vi "robot main.vi"() -> ()   [LabVIEW 2012]
uses:
  <vilib>/robotics/Starter Kit/1.0/9631 Host Interface/NI_Robotics_Starter Kit Host_9631_1.0.lvclass
  <vilib>/robotics/Starter Kit/Host Interface/NI_Robotics_Starter Kit Host.lvclass
panel:
  in  "stop":bool
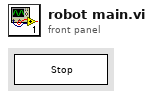
[diagram p1: front panel]
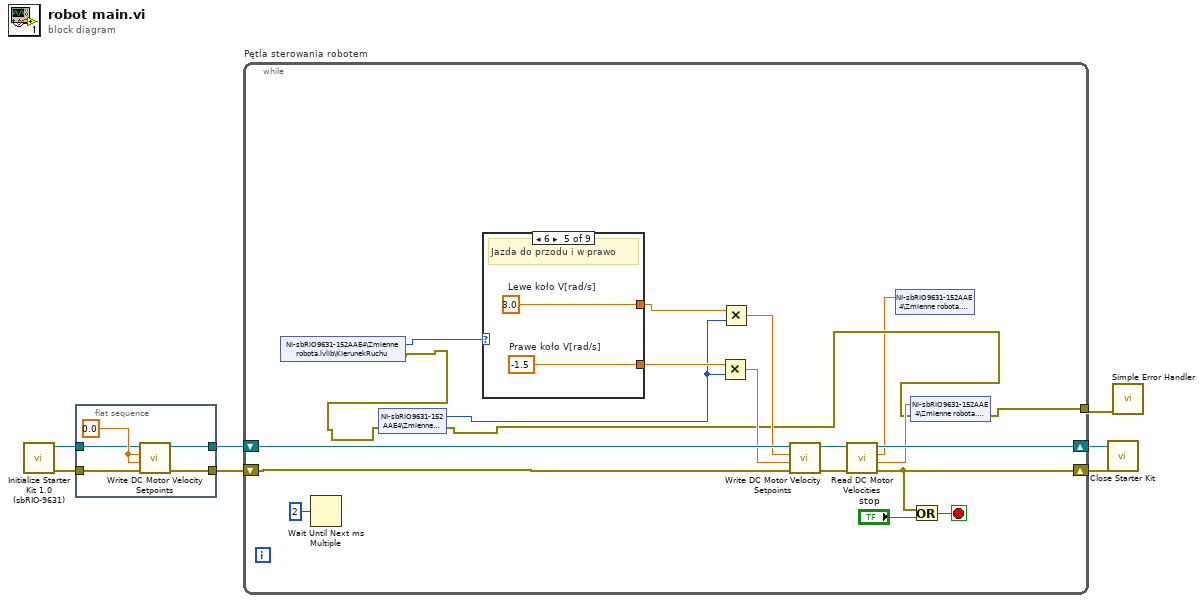
[diagram p0: block diagram]
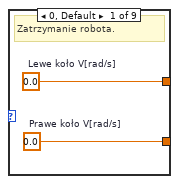
[diagram p2: hidden frame]
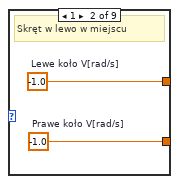
[diagram p3: hidden frame]
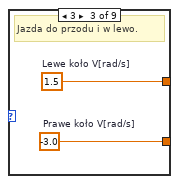
[diagram p4: hidden frame]
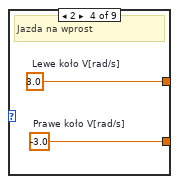
[diagram p5: hidden frame]
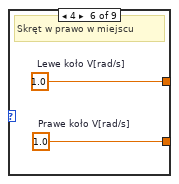
[diagram p6: hidden frame]
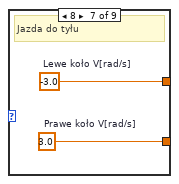
[diagram p7: hidden frame]
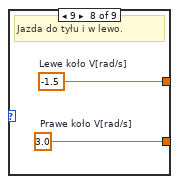
[diagram p8: hidden frame]
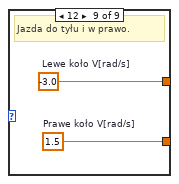
[diagram p9: hidden frame]
diagram:
  n1 = call <vilib>:"Initialize Starter Kit 1.0 (sbRIO-9631).vi"() -> ("error out"=w5:errorcluster, "FPGA starter kit host 1.0 out"=w4:refnum<class "NI_Robotics_Starter Kit Host_9631_1.0.lvclass">)  [unwired: 10 in]
  n2 = flat-sequence {
    tunnel: w4 -> [w11]
    tunnel: w5 -> [w8]
    tunnel: [w10] -> w7
    tunnel: [w9] -> w6
    frame #0 {
      w12 = 0.0 ("left ccw motor velocity (rad/s)")
      n3 = call <vilib>:"Write DC Motor Velocity Setpoints.vi"("error in (no error)"=w8, "right motor ccw velocity (rad/s)"=w12, "left motor ccw velocity (rad/s)"=w12, "starter kit host in"=w11) -> ("error out"=w9:errorcluster, "starter kit host out"=w10:refnum<class "NI_Robotics_Starter Kit Host_9631_1.0.lvclass">)  [unwired: 6 in]
    }
  }
  n4 = while "Pętla sterowania robotem" {
    shift-right: [w26] -> w2
    shift-left: w6 -> [w28]
    shift-right: [w27] -> w3
    shift-left: w7 -> [w29]
    tunnel: [w16] -> w1
    stop <- w32 stop-if-true
    n5 = shared-variable "NI-sbRIO9631-152AAE4\\Zmienne robota.lvlib\\KierunekRuchu"() -> (w19:i8, error out=w18:errorcluster)  [unwired: 1 in]
    n6 = Wait Until Next ms Multiple(millisecond multiple=u32 2) -> ()  [unwired: 1 out]
    n7 = shared-variable "NI-sbRIO9631-152AAE4\\Zmienne robota.lvlib\\Bieg"(error in=w18) -> (w17:i8, error out=w14:errorcluster)
    n8 = case shown="6" w19 {
      tunnel: [w34 w36 w38 w40 w42 w44 w46 w48 w50] -> w22
      tunnel: [w33 w35 w37 w39 w41 w43 w45 w47 w49] -> w21
      frame 0, Default {
        w33 = 0.0  # Prawe koło V[rad/s]
        w34 = 0.0  # Lewe koło V[rad/s]
        # "Zatrzymanie robota."
      }
      frame 1 {
        w35 = -1.0  # Prawe koło V[rad/s]
        w36 = -1.0  # Lewe koło V[rad/s]
        # "Skręt w lewo w miejscu"
      }
      frame 3 {
        w37 = -3.0  # Prawe koło V[rad/s]
        w38 = 1.5  # Lewe koło V[rad/s]
        # "Jazda do przodu i w lewo."
      }
      frame 2 {
        w39 = -3.0  # Prawe koło V[rad/s]
        w40 = 3.0  # Lewe koło V[rad/s]
        # "Jazda na wprost"
      }
      frame 6 {
        w41 = -1.5  # Prawe koło V[rad/s]
        w42 = 3.0  # Lewe koło V[rad/s]
        # "Jazda do przodu i w prawo"
      }
      frame 4 {
        w43 = 1.0  # Prawe koło V[rad/s]
        w44 = 1.0  # Lewe koło V[rad/s]
        # "Skręt w prawo w miejscu"
      }
      frame 8 {
        w45 = 3.0  # Prawe koło V[rad/s]
        w46 = -3.0  # Lewe koło V[rad/s]
        # "Jazda do tyłu"
      }
      frame 9 {
        w47 = 3.0  # Prawe koło V[rad/s]
        w48 = -1.5  # Lewe koło V[rad/s]
        # "Jazda do tyłu i w lewo."
      }
      frame 12 {
        w49 = 1.5  # Prawe koło V[rad/s]
        w50 = -3.0  # Lewe koło V[rad/s]
        # "Jazda do tyłu i w prawo."
      }
    }
    n9 = Multiply(x=w21, y=w17) -> (x*y=w23:dbl)
    n10 = Multiply(x=w22, y=w17) -> (x*y=w20:dbl)
    n11 = call <vilib>:"Write DC Motor Velocity Setpoints.vi"("error in (no error)"=w28, "right motor ccw velocity (rad/s)"=w23, "left motor ccw velocity (rad/s)"=w20, "starter kit host in"=w29) -> ("error out"=w24:errorcluster, "starter kit host out"=w25:refnum<class "NI_Robotics_Starter Kit Host_9631_1.0.lvclass">)  [unwired: 6 in]
    n12 = call <vilib>:"Read DC Motor Velocities.vi"("error in (no error)"=w24, "starter kit host in"=w25) -> ("error out"=w26:errorcluster, "right motor ccw velocity (rad/s)"=w15:dbl, "left motor ccw velocity (rad/s)"=w13:dbl, "starter kit host out"=w27:refnum<class "NI_Robotics_Starter Kit Host_9631_1.0.lvclass">)  [unwired: 6 in]
    n13 = shared-variable "NI-sbRIO9631-152AAE4\\Zmienne robota.lvlib\\Vl[rps]"(w13) -> ()  [unwired: 1 in, 1 out]
    n14 = shared-variable "NI-sbRIO9631-152AAE4\\Zmienne robota.lvlib\\Vr[rps]"(w15, error in=w14) -> (error out=w16:errorcluster)
    n15 = Or(x=w26, y="stop") -> (x .or. y?=w32:bool)
  }
  n16 = call-dynamic "Close Starter Kit.vi"("error in (no error)"=w2, "starter kit host in"=w3) -> ()  [unwired: 9 in, 1 out]
  n17 = call <vilib>:"Simple Error Handler.vi"("error in (no error)"=w1) -> ()  [unwired: 4 in, 5 out]
